vi "DeleteServo.vi"(8 "error in":errorcluster, 10 "Servo data":T2, 11 "Data In":T1) -> (0 "error out":errorcluster, 3 "Data Out":T1)   [LabVIEW 2023]
uses:
  controls/ServoData.ctl
  controls/UI Data.ctl
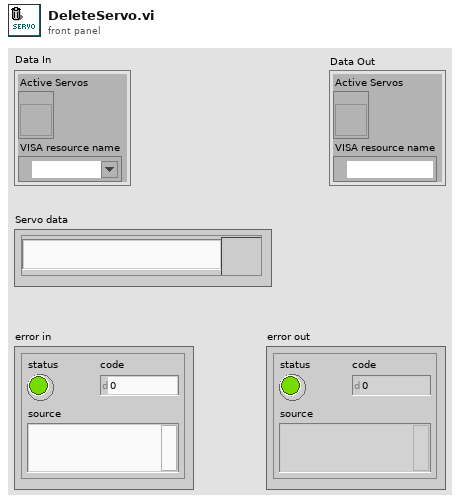
[diagram p1: front panel]
types:
  T1 = typedef "UI Data.ctl" = cluster{"Active Servos":refnum<vi>, "VISA resource name":refnum<visa-resource-name>}
  T2 = typedef "ServoData.ctl" = cluster{"Name":string, "Channel":u8, "Delete Button":bool}
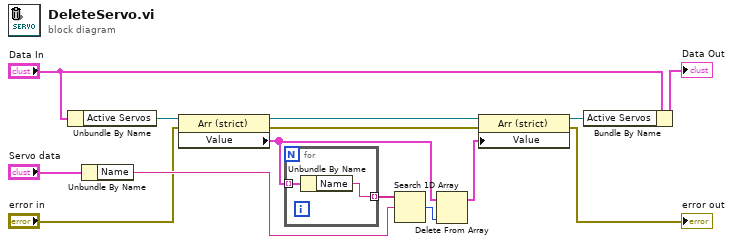
[diagram p0: block diagram]
diagram:
  n1 = Unbundle By Name("Data In") -> ("Active Servos"=w13:refnum<vi>)
  n2 = Unbundle By Name("Servo data") -> ("Name"=w4:string)
  n3 = property class="Arr (strict)"(reference=w13, error in="error in") -> (reference out=w10:refnum<vi>, error out=w2:errorcluster, "Value"=w12:T2[])
  n4 = for {
    tunnel: w12 -> [w16] mode=indexing
    tunnel: [w15] -> w11 mode=indexing
    n5 = Unbundle By Name(w16) -> ("Name"=w15:string)
  }
  n6 = Search 1D Array(1D array=w11, element=w4) -> (index of element=w14:i32)  [unwired: 1 in]
  n7 = Delete From Array(array=w12, index=w14) -> (array with subset deleted=w9:T2[])  [unwired: 1 in, 1 out]
  n8 = property class="Arr (strict)"(reference=w10, error in=w2, "Value"=w9) -> (reference out=w8:refnum<vi>, error out=→"error out":errorcluster)
  n9 = Bundle By Name(cluster="Data In", "Active Servos"=w8) -> (→"Data Out":T1)
